vi "Climb Controller Interactive Check.vi"(8 "Interactive Command in":T1={"Operation"=enum."Read Current", "Setpoint Rhino"=0.0, "Setpoint WHEELS"=0.0, "Roll"=0.0, "Pitch"=0.0, "Reset"=FALSE, "Speedy Tilt"={"Right"=TRUE, "Left"=TRUE}, "Climb"=enum."Level 1-3", "New Pos?"=FALSE, "Defense mode?"=FALSE}, 9 "Default Command":T1={"Operation"=enum."Read Current", "Setpoint Rhino"=0.0, "Setpoint WHEELS"=0.0, "Roll"=0.0, "Pitch"=0.0, "Reset"=FALSE, "Speedy Tilt"={"Right"=TRUE, "Left"=TRUE}, "Climb"=enum."Level 1-3", "New Pos?"=FALSE, "Defense mode?"=FALSE}, 11 "Buttons":cluster{"Execute Cmd":bool, "Abort Cmd":bool}) -> (1 "Interactive Command out":T1={"Operation"=enum."Read Current", "Setpoint Rhino"=0.0, "Setpoint WHEELS"=0.0, "Roll"=0.0, "Pitch"=0.0, "Reset"=FALSE, "Speedy Tilt"={"Right"=TRUE, "Left"=TRUE}, "Climb"=enum."Level 1-3", "New Pos?"=FALSE, "Defense mode?"=FALSE}, 2 "Trace String":string, 3 "Schedule":bool)   [LabVIEW 2018]
doc: "Check the Execute and Abort buttons and choose the data and trace string."
uses:
  Climb Setpoints.ctl
  Climb Operations.ctl
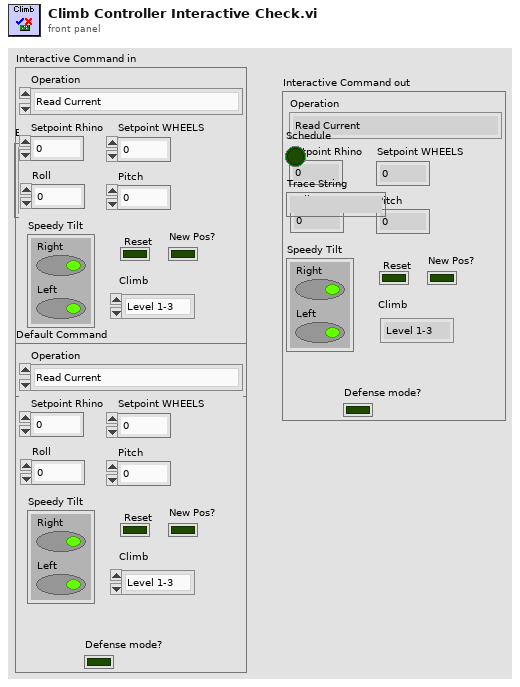
[diagram p1: front panel]
types:
  T1 = typedef "Climb Setpoints.ctl" = cluster{"Operation":T2, "Setpoint Rhino":dbl, "Setpoint WHEELS":dbl, "Roll":dbl, "Pitch":dbl, "Reset":bool, "Speedy Tilt":cluster{"Right":bool, "Left":bool}, "Climb":enum16{"Level 1-3", "Level 1-2", "Level 2-3"}, "New Pos?":bool, "Defense mode?":bool}
  T2 = typedef "Climb Operations.ctl" = enum16{"Reserve", "Read Current", "Immediate", "Ready", "Auto-Climb", "Reset/Turbo-Tilt", "Manual Climb"}
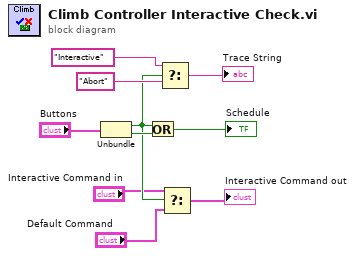
[diagram p0: block diagram]
diagram:
  n1 = Unbundle("Buttons") -> ("Execute Cmd"=w6:bool, "Abort Cmd"=w7:bool)
  n2 = Or(x=w6, y=w7) -> (x .or. y?=→"Schedule":bool)
  n3 = Select(t="Interactive", s=w6, f="Abort") -> (s? t:f=→"Trace String":string)
  n4 = Select(t="Interactive Command in", s=w6, f="Default Command") -> (s? t:f=→"Interactive Command out":T1)
